vi "Set PDOMapping.vi"(8 "error in":errorcluster, 10 "Value":refnum<class "Value.lvclass">, 11 "Object Type in":refnum<class "Object Type Base.lvclass">) -> (0 "error out":errorcluster, 3 "Object Type out":refnum<class "Object Type Base.lvclass">)   [LabVIEW 2024, in "Electronic Datasheet.lvlib" / "Object Type Base.lvclass"]
uses:
  Object Type Base.lvclass
  Value/Value.lvclass
  Object Type Base.lvclass/Object Type Base.ctl
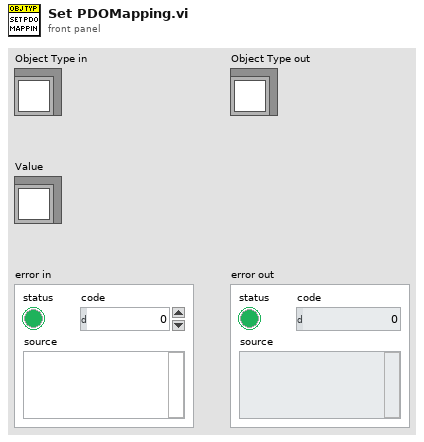
[diagram p1: front panel]
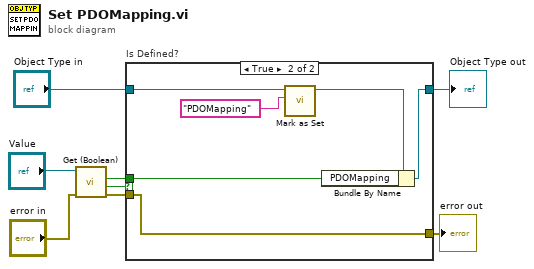
[diagram p0: block diagram]
diagram:
  n1 = call "Get (Boolean).vi"("error in"="error in", "Value in"="Value") -> ("error out"=w4:errorcluster, "Is Defined?"=w3:bool, "Value"=w2:bool)  [unwired: 6 in, 1 out]
  n2 = case "Is Defined?" shown="True" w3 {
    tunnel: "Object Type in" -> [w10 w16]
    tunnel: [w10 w15] -> w7
    tunnel: w4 -> [w9 w11]
    tunnel: w2 -> [_ w12]
    tunnel: [w9 w11] -> w1
    frame False {
    }
    frame True {
      n3 = call "Mark as Set.vi"("Field name"="PDOMapping", "Object Type in"=w16) -> ("Object Type out"=w14:refnum<class "Object Type Base.lvclass">)  [unwired: 9 in]
      n4 = Bundle By Name(cluster=w14, "PDOMapping"=w12) -> (w15:refnum<class "Object Type Base.lvclass">)
    }
  }
  "Object Type out" <- w7
  "error out" <- w1
